vi "VI-Add Event To XControl Dialog.vi"() -> ()   [LabVIEW 2015]
panel:
  in  "Event Name":string="New Event"
  out "XControl":string
  out "exit":bool
  in  "Create Event":bool
  # "XControl"
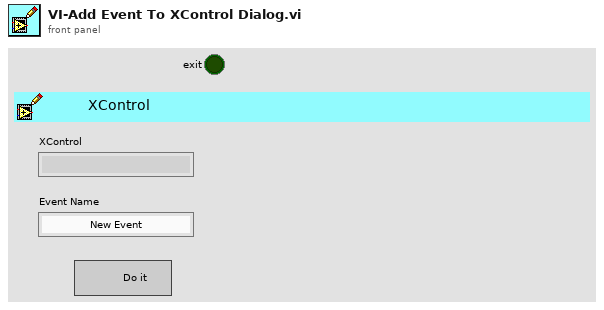
[diagram p1: front panel]
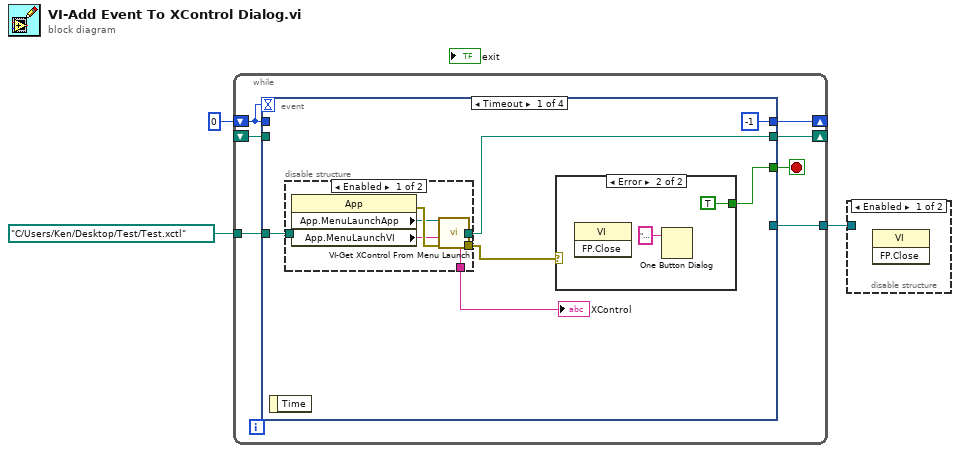
[diagram p0: block diagram]
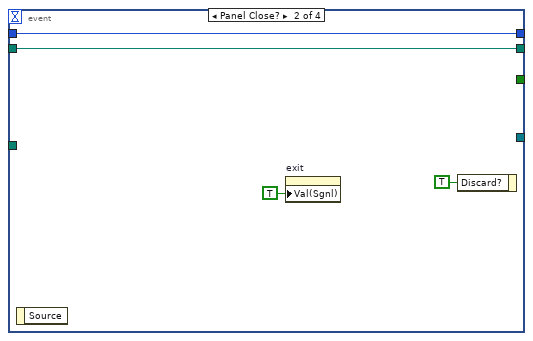
[diagram p5: hidden frame]
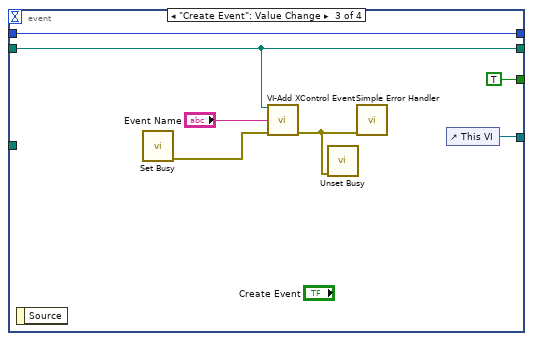
[diagram p6: hidden frame]
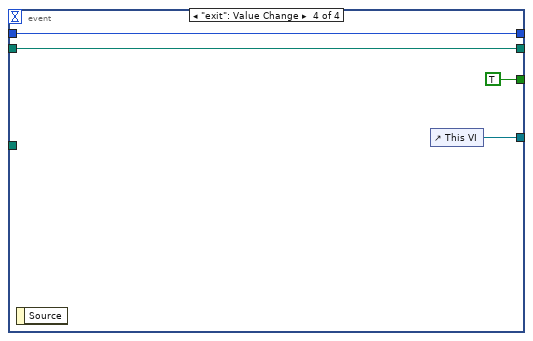
[diagram p7: hidden frame]
diagram:
  n1 = while {
    tunnel: [w10] -> w3
    shift-right: [w7] -> _
    shift-left: 0 -> [w8]
    shift-right: [w6] -> _
    shift-left: _ -> [w5]
    tunnel: path "C:/Users/Ken/Desktop/Test/Test.xctl" ("Path") -> [w4]
    stop <- w9 stop-if-true
    n2 = event shown="[0] Timeout" {
      selector: _ -> [_ _ _ _]
      dyn-events: _ -> [_ _ _ _]
      timeout: w8 -> [_ _ _ _]
      tunnel: [_ _ w35 w40] -> w10
      tunnel: [w15 _ TRUE TRUE] -> w9
      tunnel: w8 -> [_ w27 w34 w38]
      tunnel: [-1 w27 w34 w38] -> w7
      tunnel: [w13 w26 w33 w37] -> w6
      tunnel: w5 -> [_ w26 w33 w37]
      tunnel: w4 -> [w12 _ _ _]
      event Timeout {
        n3 = event-data() -> ()  [unwired: 1 in, 1 out]
        n4 = disable-structure shown="Enabled" {
          disable-tunnel: [w22 _] -> w14
          disable-tunnel: [w21 _] -> w11
          disable-tunnel: [w20 w23] -> w13
          disable-tunnel: w12 -> [_ w23]
          frame Enabled {
            n5 = property class="App"() -> (error out=w19:errorcluster, "App.MenuLaunchApp"=w17:refnum<vi>, "App.MenuLaunchVI"=w18:string)  [unwired: 2 in, 1 out]
            n6 = call "VI-Get XControl From Menu Launch.vi"("Application in"=w17, "App.MenuLaunchVI"=w18, "error in (no error)"=w19) -> ("Path"=w20:path, "Name"=w22:string, "error out"=w21:errorcluster)  [unwired: 8 in, 2 out]
          }
          frame Disabled {
          }
        }
        "XControl" <- w14
        n7 = case shown="Error" w11 {
          tunnel: [_ TRUE] -> w15
          frame No Error {
          }
          frame Error {
            n8 = invoke class="VI" method="FP.Close"() -> ()  [unwired: 3 in, 3 out]
            n9 = One Button Dialog(message="Must create a property from the menu of one of the XControl's project items.") -> ()  [unwired: 1 in, 1 out]
          }
        }
      }
      event Panel Close? {
        n10 = event-data() -> ()  [unwired: 1 in, 1 out]
        n11 = property on="exit" class="Bool (strict)"("Val(Sgnl)"=TRUE ("Value (Signaling)")) -> ()  [unwired: 2 in, 2 out]
        n12 = event-data("Discard?"=TRUE) -> ()  [unwired: 1 in, 1 out]
      }
      event "Create Event": Value Change {
        n13 = event-data() -> ()  [unwired: 1 in, 1 out]
        n14 = call <vilib>:"Set Busy.vi"() -> ("error out"=w31:errorcluster)  [unwired: 10 in, 1 out]
        n15 = call "VI-Add XControl Event.vi"("XCtl Path"=w33, "Name"="Event Name", "error in (no error)"=w31) -> ("error out"=w30:errorcluster)  [unwired: 12 in]
        n16 = call <vilib>:"Unset Busy.vi"("error in (no error)"=w30) -> ()  [unwired: 10 in, 1 out]
        n17 = call <vilib>:"Simple Error Handler.vi"("error in (no error)"=w30) -> ()  [unwired: 4 in, 5 out]
        n18 = control-ref of="This VI"() -> (w35:refnum<vi>)
      }
      event "exit": Value Change {
        n19 = event-data() -> ()  [unwired: 1 in, 1 out]
        n20 = control-ref of="This VI"() -> (w40:refnum<vi>)
      }
    }
  }
  n21 = disable-structure shown="Enabled" {
    disable-tunnel: w3 -> [_ _]
    frame Enabled {
      n22 = invoke class="VI" method="FP.Close"() -> ()  [unwired: 3 in, 3 out]
    }
    frame Disabled {
    }
  }
